vi "IRIS_set_MidPointVoltage.vi"(8 "error in (no error)":errorcluster, 10 "Channel parsed command info":T1, 11 "IRIS in":refnum<class "ISSI_Iris.lvclass">) -> (0 "error out":errorcluster, 2 "new commands":string, 3 "MKS4000b out":refnum<class "ISSI_Iris.lvclass">)   [LabVIEW 2020, in "ISSI_Iris.lvclass"]
uses:
  ISSI_Iris.lvclass
  Shared/Device Driver/channel parsed cmd cluster.ctl
  ISSI_Iris.lvclass/ISSI_Iris.ctl
  shared/CompressAndUpdate(Poly)/CompressAndUpdate(Numeric).vi
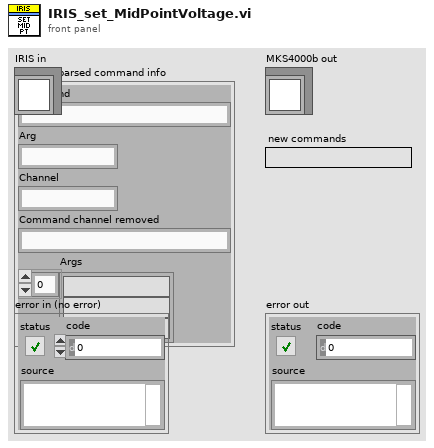
[diagram p1: front panel]
types:
  T1 = typedef "channel parsed cmd cluster.ctl" = cluster{"Command":string, "Arg":string, "Channel":string, "Command channel removed":string, "Args":string[]}
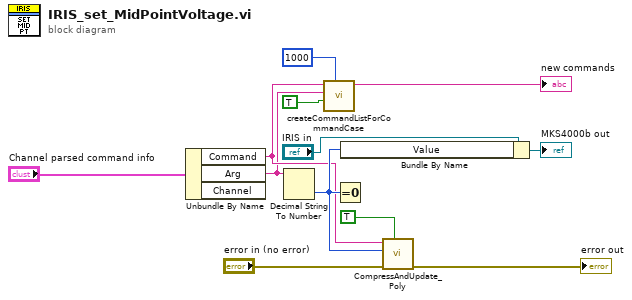
[diagram p0: block diagram]
diagram:
  n1 = Unbundle By Name("Channel parsed command info") -> ("Command"=w2:string, "Arg"=w1:string)  [unwired: 1 out]
  n2 = Decimal String To Number(string=w1) -> (number=w8:i32)  [unwired: 2 in, 1 out]
  n3 = call "createCommandListForCommandCase.vi"("timeout (optional)"=1000, "immediate Check (only once)"=TRUE, "setvalue"=w1, "command"=w2) -> ("new commands"=→"new commands":string)  [unwired: 7 in]
  n4 = Equal To 0?(x=w8) -> ()  [unwired: 1 out]
  n5 = Bundle By Name(cluster="IRIS in", "Value"=w8) -> (→"MKS4000b out":refnum<class "ISSI_Iris.lvclass">)
  n6 = call-poly "CompressAndUpdate_Poly.vi"("force CVT update (false)"=TRUE ("force CVT update"), "error in"="error in (no error)", "Numeric"=w8, "command or variable name"=w2) -> ("error out"=→"error out":errorcluster)  [unwired: 7 in]
